vi "Start.vi"(8 "error in (no error)":errorcluster, 10 "Message in":refnum<class "StartMessage.lvclass">, 11 "Cascade in":refnum<class "Cascade.lvclass">) -> (0 "error out":errorcluster, 3 "Cascade out":refnum<class "Cascade.lvclass">)   [LabVIEW 2012, in "Cascade.lvclass"]
doc: "This member function is called when the statemachine in the run.vi receives an 'start' command. It relays the message to all observers of the component.\n\nOverride this member function in your derived class if you need additional start functionality (but don't forget to call the parent method)."
uses:
  Cascade.lvclass
  <vilib>/Distrio/Murmex/StartMessage/StartMessage.lvclass
  <vilib>/Distrio/Murmex/Murmex/Murmex.lvclass
  <vilib>/Distrio/Murmex/ProceedMessage/ProceedMessage.lvclass
  Cascade.lvclass/Cascade.ctl
panel:
  # "This member function is called when the statemachine in the run.vi receives an 'start' command. It relays the message to all observers of the component.\n\nOverride this member function in your derived class if you need additional start functionality (but don't forget to call the parent method)."
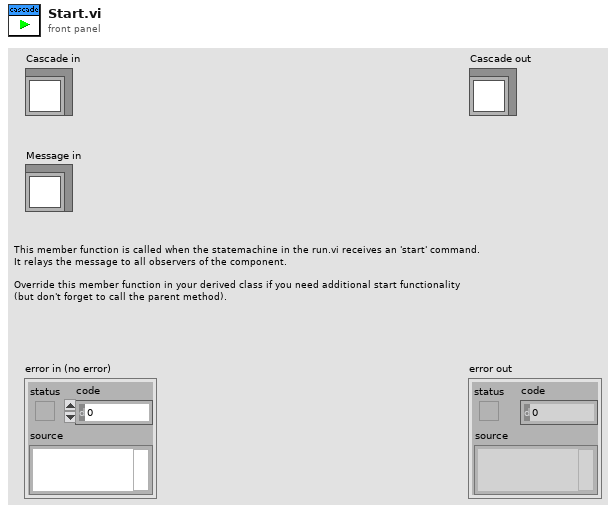
[diagram p1: front panel]
types:
  T1 = enum8{"Enabled", "Disabled", "Disabled and Grayed Out"}
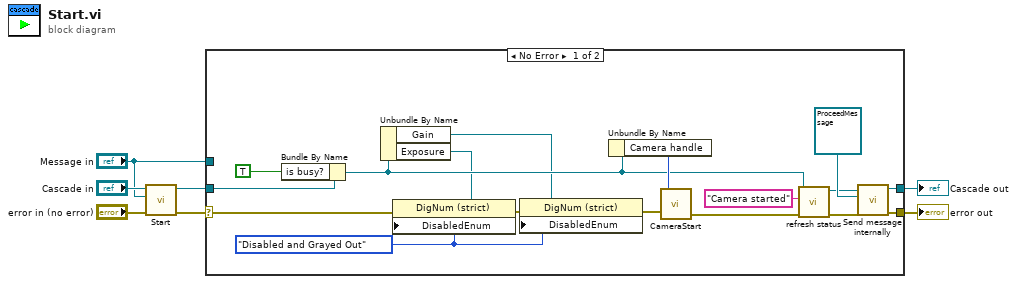
[diagram p0: block diagram]
diagram:
  n1 = call-parent "Start.vi"("error in (no error)"="error in (no error)", "Message in"="Message in", "Murmex in"="Cascade in") -> ("error out"=w6:errorcluster, "Murmex out"=w5:refnum<class "Cascade.lvclass">)  [unwired: 7 in]
  n2 = case shown="No Error" w6 {
    selector: w6 -> [w8 w26]
    tunnel: w5 -> [w20 w25]
    tunnel: [w23 w26] -> w4
    tunnel: [w22 w25] -> w1
    tunnel: "Message in" -> [_ _]
    frame No Error {
      w10 = T1."Disabled and Grayed Out" ("Disabled")
      n3 = Bundle By Name(cluster=w20, "is busy?"=TRUE ("runtime.is busy?")) -> (w15:refnum<class "Cascade.lvclass">)
      n4 = Unbundle By Name(w15) -> ("Gain"=w13:refnum<vi>, "Exposure"=w12:refnum<vi>)
      n5 = property class="DigNum (strict)"(reference=w12, error in=w8, "DisabledEnum"=w10) -> (error out=w14:errorcluster)  [unwired: 1 out]
      n6 = property class="DigNum (strict)"(reference=w13, error in=w14, "DisabledEnum"=w10) -> (error out=w11:errorcluster)  [unwired: 1 out]
      n7 = Unbundle By Name(w15) -> ("Camera handle"=w21:u32)
      n8 = call <userlib>:"CameraStart.vi"("error in"=w11, "Camera Handle"=w21) -> ("error out"=w19:errorcluster)  [unwired: 1 out]
      n9 = call-dynamic "refresh status.vi"("error in (no error)"=w19, "String In"="Camera started", "Cascade in"=w15) -> ("error out"=w18:errorcluster, "Cascade out"=w17:refnum<class "Cascade.lvclass">)  [unwired: 7 in]
      n10 = call <vilib>:"Send message internally.vi"("error in (no error)"=w18, "Message"=refnum<class "ProceedMessage.lvclass"> refnum ("ProceedMessage"), "Murmex in"=w17) -> ("error out"=w23:errorcluster, "Murmex out"=w22:refnum<class "Cascade.lvclass">)  [unwired: 7 in]
    }
    frame Error {
    }
  }
  "error out" <- w4
  "Cascade out" <- w1
